vi "Notify Event Complete.vi"(8 "error in (no error)":errorcluster, 10 "Completion Id":i64, 11 "Session in":refnum<class "Plugin Session.lvclass">) -> (0 "error out":errorcluster, 3 "Session out":refnum<class "Plugin Session.lvclass">)   [LabVIEW 2021, in "CIF_InstrumentStudio Plugin SDK.lvlib" / "Plugin Session.lvclass"]
doc: "Call this VI to notify the framework that the Project Saved event is complete. It is critical that the 'Notify Project Saved Event Complete.vi' is called in the Project Saved event so the framework does not hang"
uses:
  Plugin Session.lvclass
  Plugin Session.lvclass/Plugin Session.ctl
  Read Session Id.vi
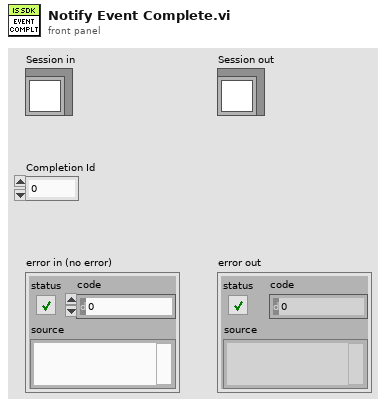
[diagram p1: front panel]
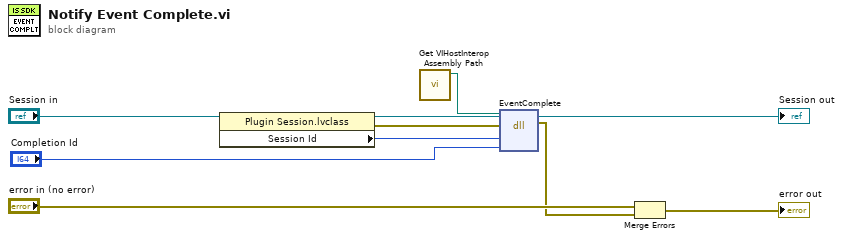
[diagram p0: block diagram]
diagram:
  n1 = property class="Plugin Session.lvclass"(reference="Session in") -> (reference out=→"Session out":refnum<class "Plugin Session.lvclass">, error out=w6:errorcluster, "Session Id"=w5:u64)  [unwired: 1 in]
  n2 = call "Get VIHostInterop Assembly Path.vi"() -> ("VIHost.Interop Assembly"=w1:path)  [unwired: 11 in]
  n3 = dll-call lib="C:/ASW/Source/InstrumentStudio/IFDistribution/VIHostPanel/objects/export/targets/win64U/x64/msvc-14.0/debug/NationalInstruments.VIHost.Interop.dll" fn="EventComplete"(path in=w1, error in=w6, "hostId"=w5, "completionId"="Completion Id") -> (error out=w3:errorcluster)  [unwired: 4 in, 1 out]
  n4 = Merge Errors("error in (no error)", w3) -> (→"error out":errorcluster)
